vi "Heater.vi"() -> ()   [LabVIEW 2012]
uses:
  <vilib>/rvi/eio/common/nirviEmuTemplateMethod_errors.vi
  <vilib>/rvi/Emulation/niFpgaSctlEmulationGetInTimedLoop.vi
  <vilib>/rvi/Emulation/niFpgaSctlEmulationGlobalWrite.vi
  <vilib>/eio/EIONode/EIONode.xnode
  <vilib>/addons/control/pid/fpga.llb/XNode/niFpgaPID.xnode
panel:
  out "Temperature":i16
  in  "tenperature  factor":i16
  out "Input":i16
  in  "Output":i16
  in  "setpoint":fxp<+/-,16,16>
  in  "PID gains":T1={"proportional gain (Kc)"=1.0, "integral gain (Kc*Ts/Ti)"=1.66796875, "derivative gain (Kc*Td/Ts)"=0.0}
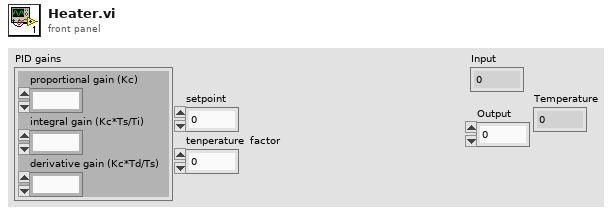
[diagram p1: front panel]
types:
  T1 = cluster{"proportional gain (Kc)":fxp<+/-,16,8>, "integral gain (Kc*Ts/Ti)":fxp<+/-,16,8>, "derivative gain (Kc*Td/Ts)":fxp<+/-,16,8>}
  T2 = cluster{"proportional gain (Kc)":i16, "integral gain (Kc*Ts/Ti)":i16, "derivative gain (Kc*Td/Ts)":i16}
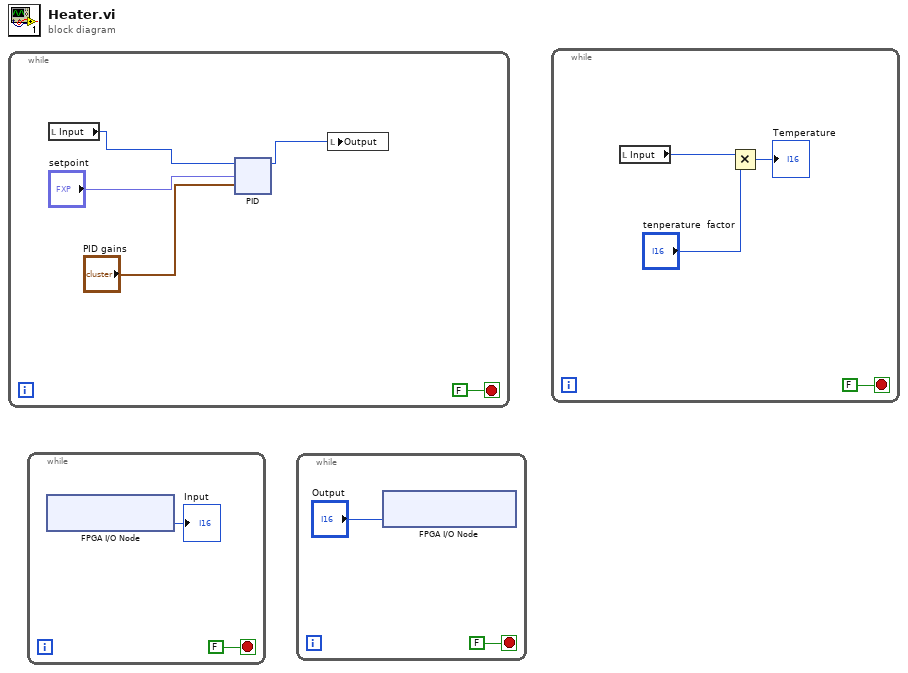
[diagram p0: block diagram]
diagram:
  n1 = while {
    stop <- FALSE stop-if-true
    n2 = local read "Input"() -> (w1:i16)
    n3 = xnode "PID"("process variable"=w1, "setpoint"="setpoint", "PID gains"="PID gains") -> ("output"=w2:i16)  [unwired: 2 in]
    n4 = local write "Output"(w2) -> ()
  }
  n5 = while {
    stop <- FALSE stop-if-true
    n6 = xnode "FPGA I/O Node"() -> ("Connector0/AI1"=→"Input":i16)  [unwired: 1 in, 1 out]
  }
  n7 = while {
    stop <- FALSE stop-if-true
    n8 = xnode "FPGA I/O Node"("Connector0/AO1"="Output") -> ()  [unwired: 1 in, 1 out]
  }
  n9 = while {
    stop <- FALSE stop-if-true
    n10 = local read "Input"() -> (w41:i16)
    n11 = Multiply(x=w41, y="tenperature  factor") -> (x*y=→"Temperature":i16)
  }
